vi "MIPI RFFE Read Waveform.vi"(0 "Data":T2 {"Register" max=31 format="%.0x"; "Slave Address" max=15 format="%.0x"}, 2 "Readback Speed":enum16{"Full Speed", "Half Speed"}(ring), 5 "Configuratation":T3={"Samples to Allocate"=10000, "Oversample Factor"=1, "Clock Channel"=enum."0", "Data Channel"=enum."1"} {"Oversample Factor" min=1 max=254; "Samples to Allocate" min=1}, 11 "error in (no error)":errorcluster) -> (6 "Waveform Graph":digitalwaveform(graph), 8 "Compare Bits Out":T1[](array[typedef]) {"Expected Value(s)" format="%.0x"}, 15 "error out":errorcluster)   [LabVIEW 2013]
uses:
  Ctrls/Configuration.ctl
  Ctrls/ClockDataChannels.ctl
  Ctrls/RegReadWrite.ctl
  Ctrls/ReadInfo.ctl
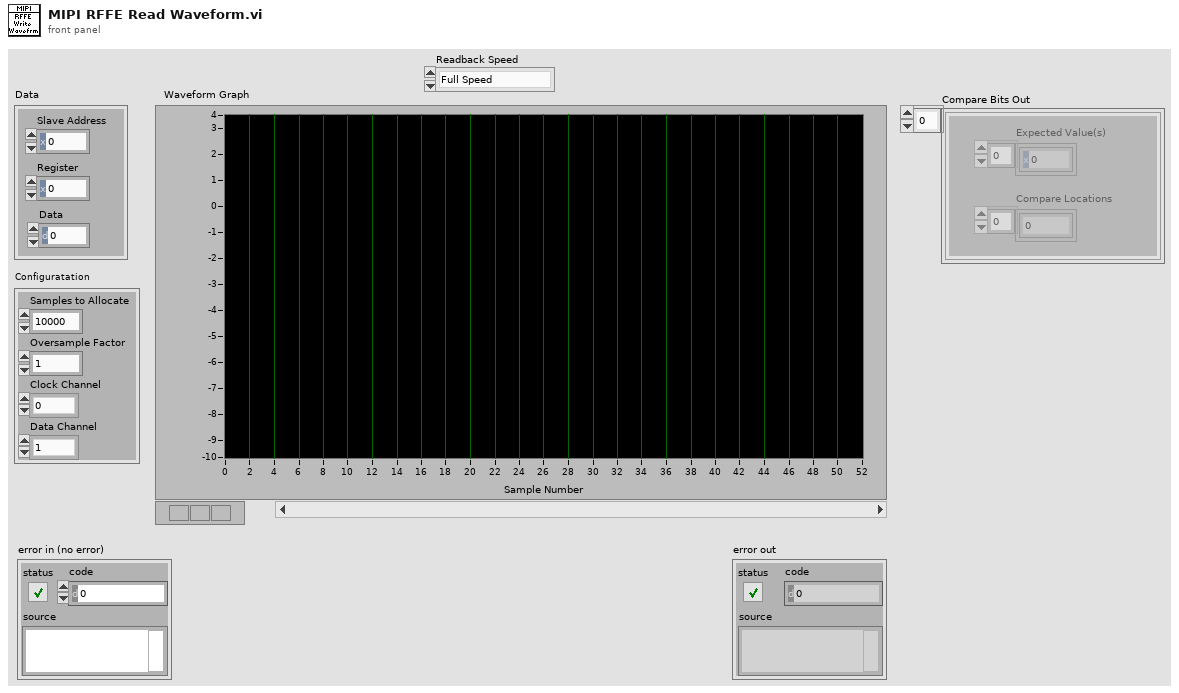
[diagram p1: front panel]
types:
  T1 = typedef "ReadInfo.ctl" = cluster{"Expected Value(s)":u8[], "Compare Locations":u32[]}
  T2 = typedef "RegReadWrite.ctl" = cluster{"Slave Address":u8, "Register":u8, "Data":u8}
  T3 = typedef "Configuration.ctl" = cluster{"Samples to Allocate":i32, "Oversample Factor":u8, "Clock Channel":T4, "Data Channel":T4}
  T4 = typedef "ClockDataChannels.ctl" = enum16{"0", "1"}
  T5 = typedef "RFFE_Data.ctl" = cluster{"Clock Channel":T4, "Data Channel":T4, "Oversample Factor":u8, "Zero Array":u8[], "One Array":u8[], "Z Array ":u8[], "H Array":u8[], "L Array":u8[], "X Array":u8[], "Toggle (high to low)":u8[]}
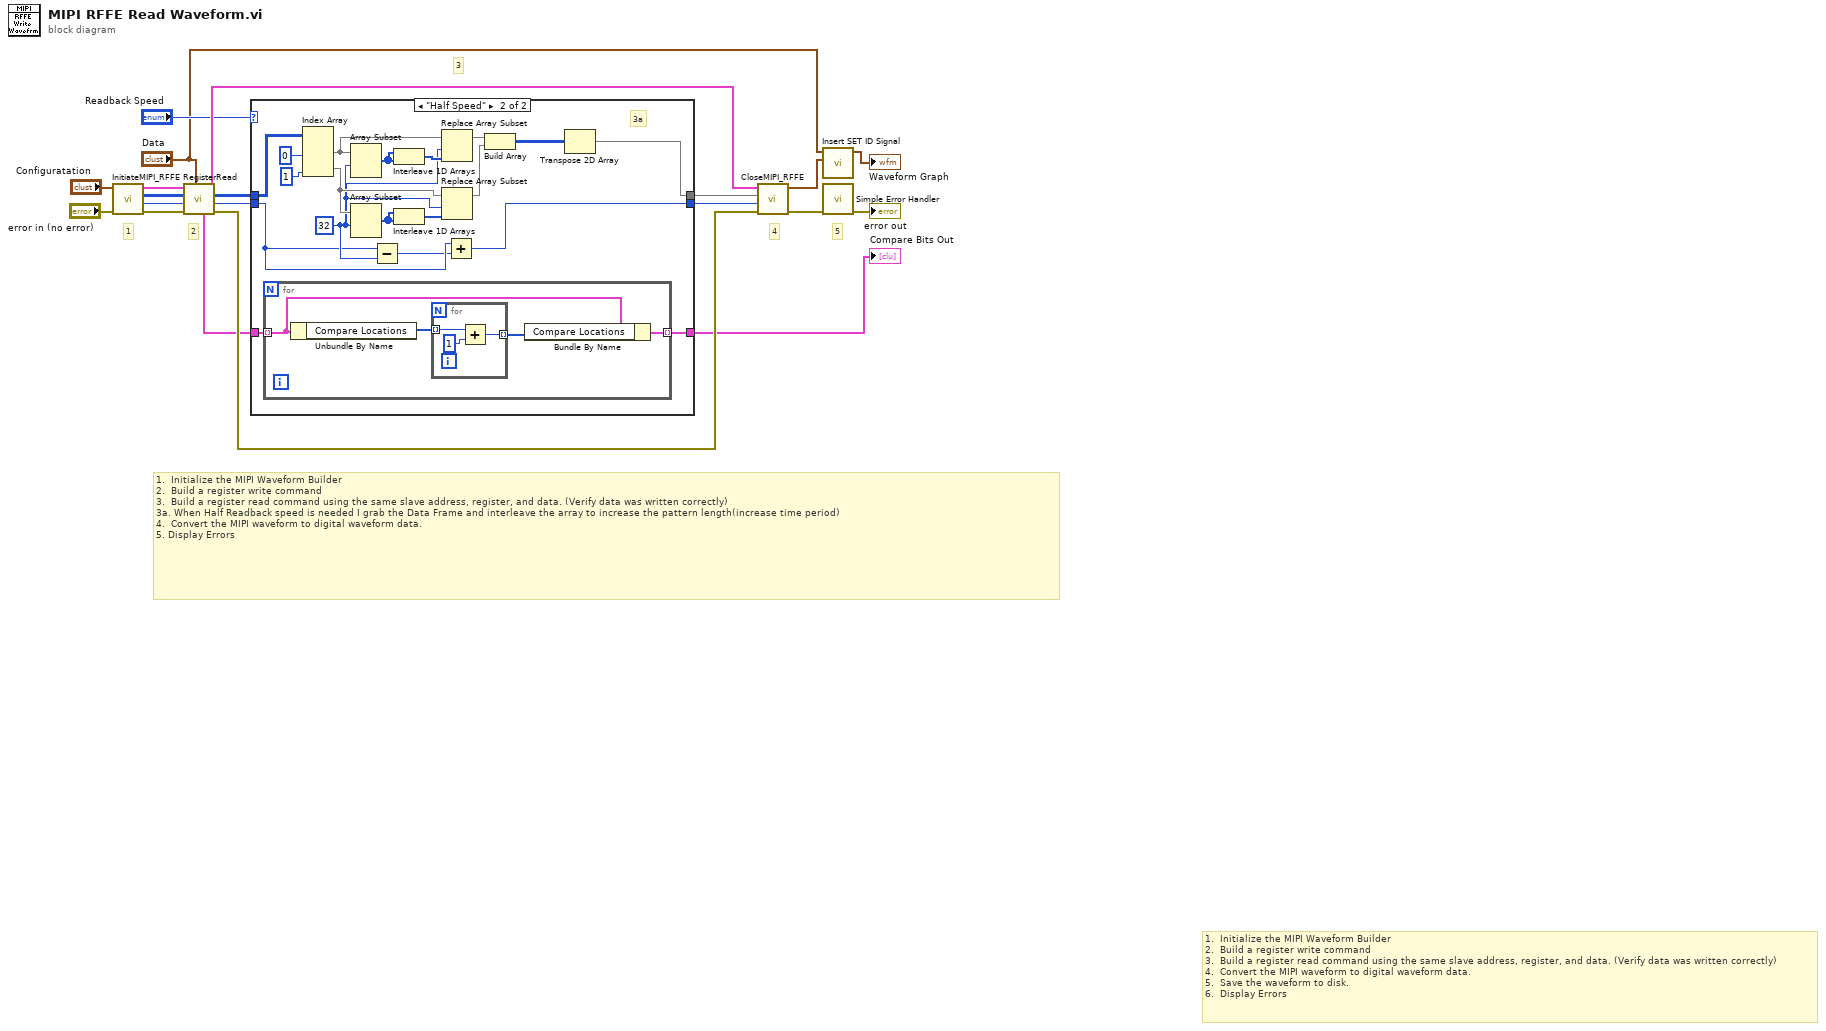
[diagram p0: block diagram]
diagram:
  # "3"
  # "1.  Initialize the MIPI Waveform Builder\n2.  Build a register write command\n3.  Build a register read command using the same slave address, register, and data. (Verify data was written correctly)\n3a. When Half Readback speed is needed I grab the Data Frame and interleave the array to increase the pattern length(increase time period)\n4.  Convert the MIPI waveform to digital waveform data.\n5. Display Errors"
  # "5"
  # "1.  Initialize the MIPI Waveform Builder\n2.  Build a register write command\n3.  Build a register read command using the same slave address, register, and data. (Verify data was written correctly)\n4.  Convert the MIPI waveform to digital waveform data.\n5.  Save the waveform to disk.\n6.  Display Errors"
  # "4"
  # "2"
  # "1"
  n1 = call "InitiateMIPI_RFFE.vi"("error in (no error)"="error in (no error)", "Configuratation In"="Configuratation") -> ("error out"=w13:errorcluster, "Number of Samples Out"=w14:i32, "Data Array"=w15:u8[][], "RFFE_Data"=w16:T5)  [unwired: 6 in]
  n2 = call "RegisterRead.vi"("Register Read/Write"="Data", "error in (no error)"=w13, "Number of Samples In"=w14, "Data Array"=w15, "RFFE_Data In"=w16) -> ("error out"=w12:errorcluster, "Number of Samples Out out"=w7:i32, "Data Array Out"=w9:u8[][], "RFFE_Data Out"=w11:T5, "Compare Bits Out"=w5:T1[])  [unwired: 2 in]
  n3 = case shown="\"Half Speed\"" "Readback Speed" {
    tunnel: w9 -> [w23 w31]
    tunnel: [w23 w30] -> w8
    tunnel: w7 -> [w22 w28]
    tunnel: [w22 w26] -> w6
    tunnel: w5 -> [w21 w25]
    tunnel: [w21 w24] -> w4
    frame "Full Speed", Default {
    }
    frame "Half Speed" {
      w29 = 32 ("index")
      # "3a"
      n4 = for {
        tunnel: w25 -> [w45] mode=indexing
        tunnel: [w43] -> w24 mode=indexing
        n5 = Unbundle By Name(w45) -> ("Compare Locations"=w46:u32[])
        n6 = for {
          tunnel: w46 -> [w49] mode=indexing
          tunnel: [w47] -> w44 mode=indexing
          n7 = Add(x=w49, y=u32 1) -> (x+y=w47:u32)
        }
        n8 = Bundle By Name(cluster=w45, "Compare Locations"=w44) -> (w43:T1)
      }
      n9 = Index Array(array=w31, index (col) #1=0 ("index (row)"), index (col) #2=1 ("index (row)")) -> (element #1=w36:u8[], element #2=w41:u8[])  [unwired: 2 in]
      n10 = Array Subset(array=w36, index=w29) -> (w32:u8[])  [unwired: 1 in]
      n11 = Array Subset(array=w41, index=w29) -> (w33:u8[])  [unwired: 1 in]
      n12 = Subtract(x=w28, y=w29) -> (x-y=w27:i32)
      n13 = Interleave 1D Arrays(w32, w32) -> (w42:u8[])
      n14 = Interleave 1D Arrays(w33, w33) -> (w37:u8[])
      n15 = Replace Array Subset(array=w36, new element=w42, index=w29) -> (w38:u8[])
      n16 = Replace Array Subset(array=w41, new element=w37, index=w29) -> (w40:u8[])
      n17 = Add(x=w28, y=w27) -> (x+y=w26:i32)
      n18 = Build Array(w38, w40) -> (w39:u8[][])
      n19 = Transpose 2D Array(2D array=w39) -> (transposed array=w30:u8[][])
    }
  }
  "Compare Bits Out" <- w4
  n20 = call "CloseMIPI_RFFE.vi"("error in (no error)"=w12, "Number of Samples"=w6, "Data Array"=w8, "RFFE_Data"=w11) -> ("error out"=w19:errorcluster, "Digital Waveform"=w3:digitalwaveform)  [unwired: 6 in]
  n21 = call "Insert SET ID Signal.vi"("Digital Waveform Graph"=w3, "Data"="Data") -> ("Digital Waveform Graph 2"=→"Waveform Graph":digitalwaveform)  [unwired: 9 in]
  n22 = call <vilib>:"Simple Error Handler.vi"("error in (no error)"=w19) -> ("error out"=→"error out":errorcluster)  [unwired: 4 in, 4 out]
